vi "SCPI Encode.vi"(0 "Command [VERB]":string, 7 "Arguments [NOUNS]":string[](array[string])) -> (6 "Command String":string)   [LabVIEW 2016, in "SCPI.lvclass"]
uses:
  SCPI.lvclass
panel:
  # "Example:\nsetConfig >> Sys >> Time >> hh:mm:ss\nsetConfig >> Sys >> Date >> yyyy:mm:dd\nsetSignal >> Magnet >> Target Current >> float (-170 to +170)\n\nInspiration: SCPI:\n<VERB>:<NOUN>:<NOUN>"
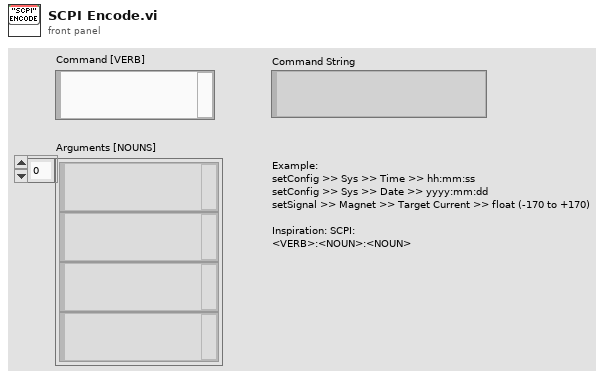
[diagram p1: front panel]
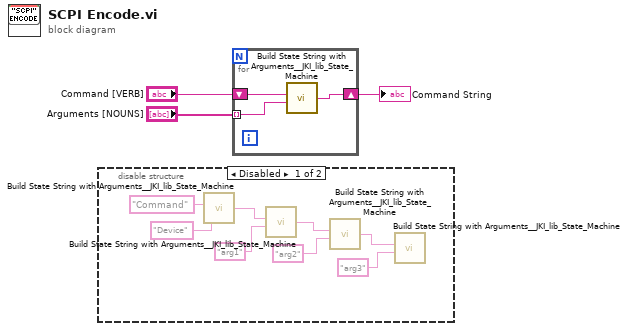
[diagram p0: block diagram]
diagram:
  n1 = disable-structure shown="Disabled" {
    frame Disabled {
      n2 = call <vilib>:"Build State String with Arguments__JKI_lib_State_Machine.vi"("Arguments (\"\")"="Device" ("Arguments (\"\")"), "State"="Command") -> ("State with Arguments"=w11:string)  [unwired: 4 in]
      n3 = call <vilib>:"Build State String with Arguments__JKI_lib_State_Machine.vi"("Arguments (\"\")"="arg1" ("Arguments (\"\")"), "State"=w11) -> ("State with Arguments"=w10:string)  [unwired: 4 in]
      n4 = call <vilib>:"Build State String with Arguments__JKI_lib_State_Machine.vi"("Arguments (\"\")"="arg2" ("Arguments (\"\")"), "State"=w10) -> ("State with Arguments"=w9:string)  [unwired: 4 in]
      n5 = call <vilib>:"Build State String with Arguments__JKI_lib_State_Machine.vi"("Arguments (\"\")"="arg3" ("Arguments (\"\")"), "State"=w9) -> ()  [unwired: 4 in, 1 out]
    }
    frame Enabled {
    }
  }
  n6 = for {
    shift-right: [w12] -> w1
    shift-left: "Command [VERB]" -> [w14]
    tunnel: "Arguments [NOUNS]" -> [w13] mode=indexing
    n7 = call <vilib>:"Build State String with Arguments__JKI_lib_State_Machine.vi"("Arguments (\"\")"=w13, "State"=w14) -> ("State with Arguments"=w12:string)  [unwired: 4 in]
  }
  "Command String" <- w1
